vi "Acorrection(SubVI).vi"(8 "length":i32=37, 9 "index":i32=44, 10 "Lambda":dbl[](array[numeric]), 11 "Ain":dbl[](array[numeric])) -> (2 "slope":dbl, 3 "Aout":dbl[](array[numeric]))   [LabVIEW 2019]
uses:
  <vilib>/Analysis/NI_AALPro.lvlib
panel:
  out "intercept":dbl
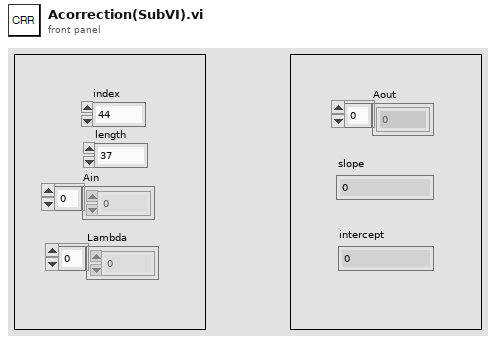
[diagram p1: front panel]
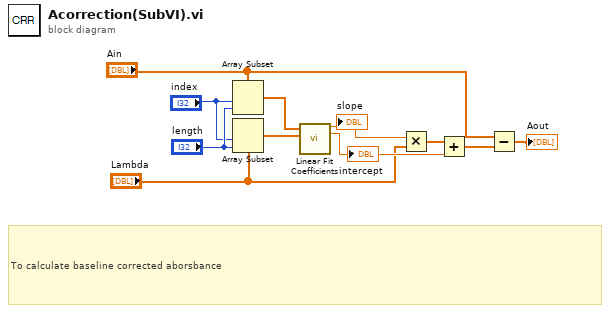
[diagram p0: block diagram]
diagram:
  # "To calculate baseline corrected aborsbance"
  n1 = Array Subset(array="Ain", index="index", length="length") -> (w7:dbl[])
  n2 = Array Subset(array="Lambda", index="index", length="length") -> (w6:dbl[])
  n3 = call <vilib>:"Linear Fit Coefficients.vi"("Y"=w7, "X"=w6) -> ("slope"=w5:dbl, "intercept"=w4:dbl)  [unwired: 11 in, 1 out]
  "slope" <- w5
  "intercept" <- w4
  n4 = Multiply(x=w5, y="Lambda") -> (x*y=w11:dbl[])
  n5 = Add(x=w11, y=w4) -> (x+y=w10:dbl[])
  n6 = Subtract(x="Ain", y=w10) -> (x-y=→"Aout":dbl[])
